vi "Init_HTTP.vi"(8 "error in (no error)":errorcluster, 11 "ByteGSAPIBase in":refnum<class "ByteGSAPIBase.lvclass">) -> (0 "error out":errorcluster, 3 "ByteGSAPIBase out":refnum<class "ByteGSAPIBase.lvclass">)   [LabVIEW 2019, in "ByteGSWebAPI.lvlib" / "ByteGSAPIBase.lvclass"]
doc: "Apre una nuova connessione HTTP e setta il content type a \"application/json\""
uses:
  ByteGSAPIBase.lvclass
  ByteGSAPIBase.lvclass/ByteGSAPIBase.ctl
  <vilib>/httpClient/LabVIEWHTTPClient.lvlib
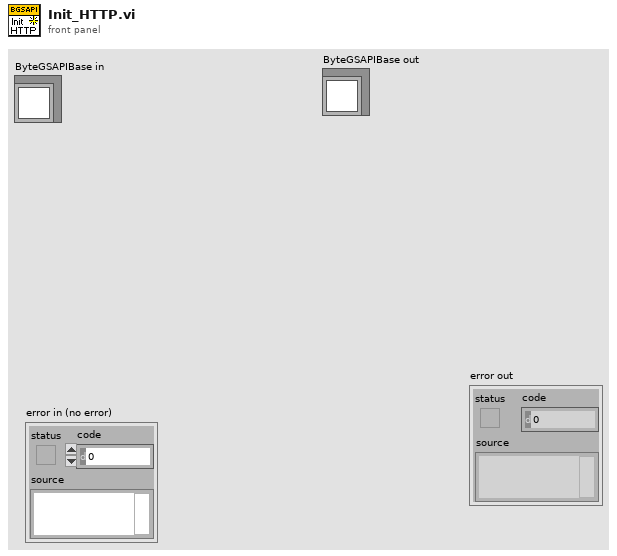
[diagram p1: front panel]
types:
  T1 = typedef "LabVIEWHTTPClient.lvlib/ClientHandle.ctl" = refnum<k1>
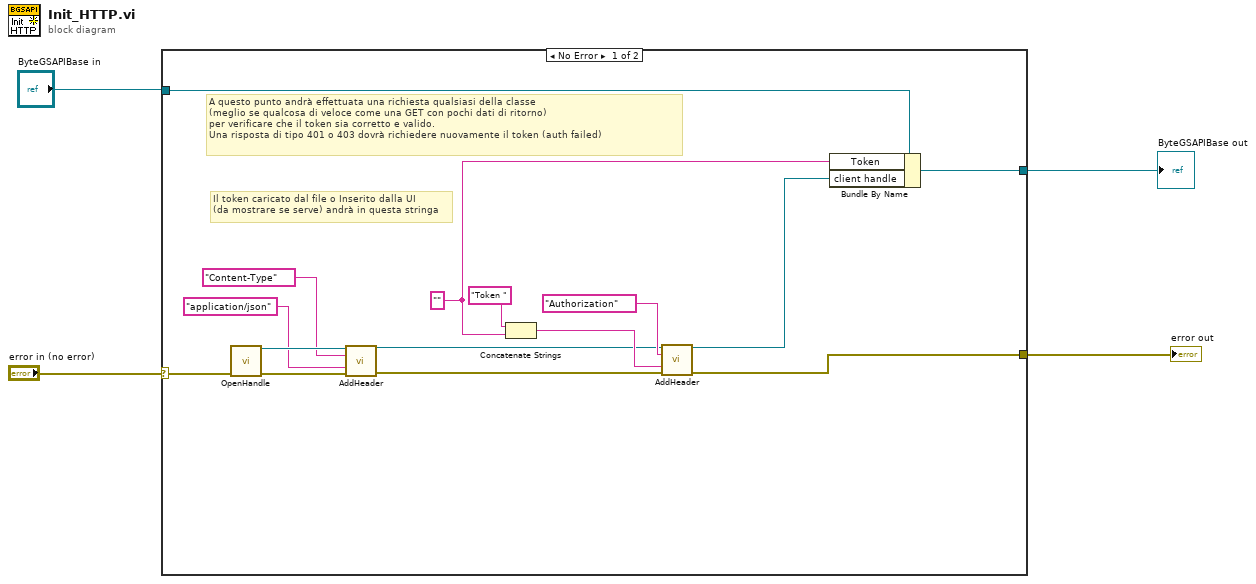
[diagram p0: block diagram]
diagram:
  n1 = case shown="No Error" "error in (no error)" {
    selector: "error in (no error)" -> [w14 w21]
    tunnel: [w6 w21] -> w3
    tunnel: [w15 w20] -> w1
    tunnel: "ByteGSAPIBase in" -> [w8 w20]
    frame No Error {
      w7 = ""
      # "A questo punto andrà effettuata una richiesta qualsiasi della classe\n(meglio se qualcosa di veloce come una GET con pochi dati di ritorno)\nper verificare che il token sia corretto e valido.\nUna risposta di tipo 401 o 403 dovrà richiedere nuovamente il token (auth failed)"
      # "Il token caricato dal file o Inserito dalla UI\n(da mostrare se serve) andrà in questa stringa"
      n2 = call <vilib>:"OpenHandle.vi"("error in (no error)"=w14) -> ("client handle out"=w18:T1, "error out"=w19:errorcluster)  [unwired: 13 in]
      n3 = call <vilib>:"AddHeader.vi"("client handle"=w18, "header"="Content-Type", "value"="application/json", "error in (no error)"=w19) -> ("client handle out"=w10:T1, "error out"=w9:errorcluster)  [unwired: 10 in]
      n4 = Concatenate Strings("Token " ("string"), w7) -> (w12:string)
      n5 = call <vilib>:"AddHeader.vi"("client handle"=w10, "header"="Authorization", "value"=w12, "error in (no error)"=w9) -> ("client handle out"=w5:T1, "error out"=w6:errorcluster)  [unwired: 10 in]
      n6 = Bundle By Name(cluster=w8, "Token"=w7, "client handle"=w5) -> (w15:refnum<class "ByteGSAPIBase.lvclass">)
    }
    frame Error {
    }
  }
  "error out" <- w3
  "ByteGSAPIBase out" <- w1
